vi "HIOKI PW3390 Conf Scale.vi"(0 "VISA Resource":refnum<visa-resource-name>, 1 "Set/Query (F: Set)":bool, 2 "CH (1)":i32=1 min=1 max=4, 5 "CT Rate (1: OFF)":dbl=1.0 min=0.01 max=9999.99 format="%.2f", 7 "VT Rate (1: OFF)":dbl=1.0 min=0.01 max=9999.99 format="%.2f", 11 "error in (no error)":errorcluster, 12 "OPC query (T: ON)":bool=TRUE, 13 "Error Out (F: Off)":bool) -> (4 "VISA Resource out":refnum<visa-resource-name>, 6 "CT Rate out":dbl=1.0 format="%.2f", 8 "VT Rate out":dbl=1.0 format="%.2f", 15 "error out":errorcluster)   [LabVIEW 2009]
doc: "Sets and reads the CT, VT rate.\n\nSet/Query\n Set: Send the setting commands for the device.\n Query: Query the setting of the device.\n\nCT Rate\n Sets the CT ratio of the specified channel.\n Input Range: 0. 01-9999.99\nVT Rate\n Sets the VT ratio of the specified channel.\n Input Range: 0. 01-9999.99\nIt is limited at VT * CT <= 1.0E+06.\n\n<B>Note</B>\nThe setting for CT, VT ratio OFF is 1. The query response for OFF is 1. The settings for other channels in the measurement line combination will be changed. Specify the starting channel in the channel combination."
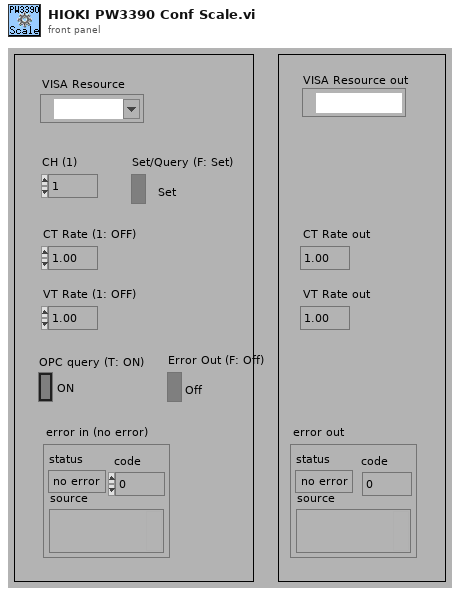
[diagram p1: front panel]
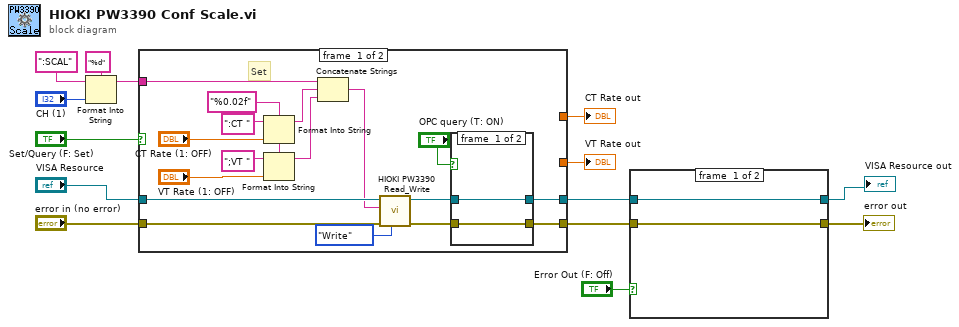
[diagram p0: block diagram]
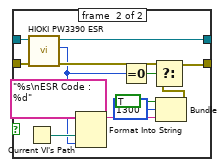
[diagram p2: hidden frame]
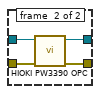
[diagram p3: hidden frame]
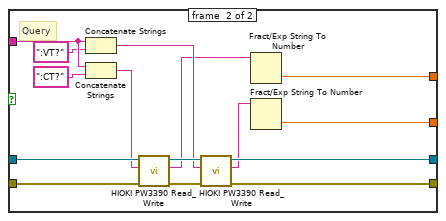
[diagram p4: hidden frame]
diagram:
  n1 = Format Into String(format string="%d", initial string=":SCAL", "CH (1)") -> (resulting string=w3:string)  [unwired: 1 in, 1 out]
  n2 = case shown="FALSE" "Set/Query (F: Set)" {
    tunnel: "error in (no error)" -> [w30 w47]
    tunnel: [w15 w50] -> w11
    tunnel: "VISA Resource" -> [w31 w48]
    tunnel: [w16 w49] -> w10
    tunnel: [_ w39] -> w8
    tunnel: [_ w38] -> w7
    tunnel: w3 -> [w22 w46]
    frame #0 {
      w21 = "%0.02f"
      # "Set"
      n3 = Format Into String(format string=w21, initial string=":CT ", "CT Rate (1: OFF)") -> (resulting string=w24:string)  [unwired: 1 in, 1 out]
      n4 = Format Into String(format string=w21, initial string=";VT ", "VT Rate (1: OFF)") -> (resulting string=w20:string)  [unwired: 1 in, 1 out]
      n5 = Concatenate Strings(w22, w24, w20) -> (w23:string)
      n6 = call <instrlib>:"HIOKI PW3390 Read_Write.vi"("Read/Write"=enum16{"Read", "Write"}."Write", "error in (no error)"=w30, "data in"=w23, "VISA Resource"=w31) -> ("error out"=w17:errorcluster, "VISA Resource out"=w18:refnum<visa-resource-name>)  [unwired: 5 in, 1 out]
      n7 = case shown="TRUE" "OPC query (T: ON)" {
        tunnel: [w33 w37] -> w16
        tunnel: [w32 w36] -> w15
        tunnel: w18 -> [w33 w35]
        tunnel: w17 -> [w32 w34]
        frame #0 {
        }
        frame #1 {
          n8 = call <instrlib>:"HIOKI PW3390 OPC.vi"("error in (no error)"=w34, "VISA Resource"=w35) -> ("error out"=w36:errorcluster, "VISA Resource out"=w37:refnum<visa-resource-name>)  [unwired: 7 in, 1 out]
        }
      }
    }
    frame #1 {
      # "Query"
      n9 = Concatenate Strings(w46, ":VT?" ("文字列")) -> (w45:string)
      n10 = Concatenate Strings(w46, ":CT?" ("文字列")) -> (w44:string)
      n11 = call <instrlib>:"HIOKI PW3390 Read_Write.vi"("error in (no error)"=w47, "data in"=w44, "VISA Resource"=w48) -> ("error out"=w52:errorcluster, "data out"=w41:string, "VISA Resource out"=w51:refnum<visa-resource-name>)  [unwired: 6 in]
      n12 = call <instrlib>:"HIOKI PW3390 Read_Write.vi"("error in (no error)"=w52, "data in"=w45, "VISA Resource"=w51) -> ("error out"=w50:errorcluster, "data out"=w40:string, "VISA Resource out"=w49:refnum<visa-resource-name>)  [unwired: 6 in]
      n13 = Fract/Exp String To Number(string=w41) -> (number=w38:dbl)  [unwired: 3 in, 1 out]
      n14 = Fract/Exp String To Number(string=w40) -> (number=w39:dbl)  [unwired: 3 in, 1 out]
    }
  }
  "CT Rate out" <- w7
  "VT Rate out" <- w8
  n15 = case shown="TRUE" "Error Out (F: Off)" {
    tunnel: w10 -> [w54 w67]
    tunnel: w11 -> [w53 w66]
    tunnel: [w53 w56] -> w9
    tunnel: [w54 w65] -> w1
    frame #0 {
    }
    frame #1 {
      n16 = Current VI's Path() -> (path=w63:path)
      n17 = call <instrlib>:"HIOKI PW3390 ESR.vi"("error in (no error)"=w66, "VISA Resource"=w67) -> ("error out"=w57:errorcluster, "Output Value"=w55:u8, "VISA Resource out"=w65:refnum<visa-resource-name>)  [unwired: 6 in, 1 out]
      n18 = Format Into String(format string="%s\nESR Code : %d", w63, w55) -> (resulting string=w59:string)  [unwired: 2 in, 1 out]
      n19 = Equal To 0?(x=w55) -> (x = 0?=w64:bool)
      n20 = Bundle("status"=TRUE, "code"=1300, w59) -> (w58:cluster{"status":bool, "code":i32, string})  [unwired: 1 in]
      n21 = Select(t=w57, s=w64, f=w58) -> (s? t:f=w56:errorcluster)
    }
  }
  "error out" <- w9
  "VISA Resource out" <- w1
